vi "From String Array.vi"(8 "error in (no error)":errorcluster, 9 "String Array":string[](array[string]), 11 "Wait On Integer Step Config in":refnum<class "Wait On Integer Config.lvclass">) -> (0 "error out":errorcluster, 1 "Elements Left":string[](array[string]), 2 "Version":string, 3 "Wait On Integer Step Config out":refnum<class "Wait On Integer Config.lvclass">)   [LabVIEW 2018, in "Wait On Integer Config.lvclass"]
uses:
  Wait On Integer Config.lvclass
  <vilib>/NI/Tag Bus/tag/Data Type.ctl
  <vilib>/NI/Tag Bus Module Framework/channel/channel classification.ctl
  Wait On Integer Config.lvclass/Wait On Integer Config.ctl
  classes/Step/Config/Step Config.lvclass
  <vilib>/NI/Tag Bus Module Framework/channel/TBM channel.lvclass
  <vilib>/NI/Tag Bus/tag/tag descriptor.lvclass
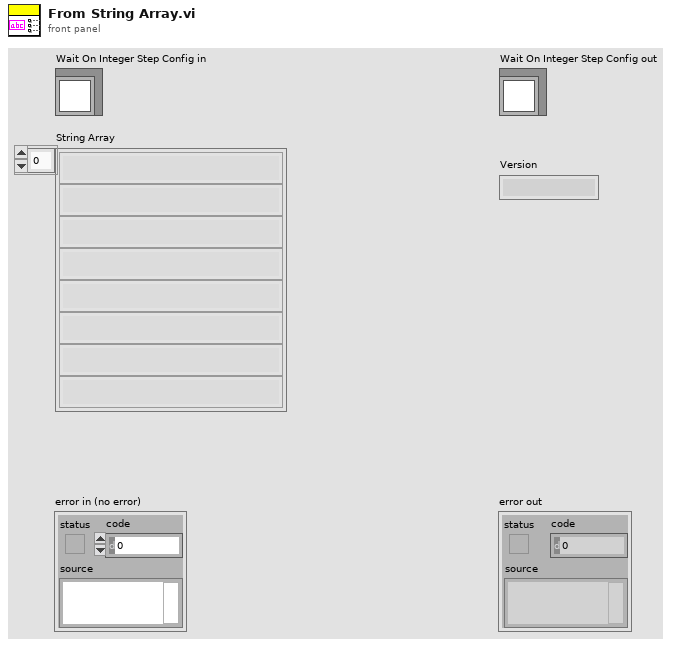
[diagram p1: front panel]
types:
  T1 = typedef "TBM channel.lvclass/channel classification.ctl" = enum16{"input data", "output data", "processing parameter", "processing result"}
  T2 = typedef "tag bus.lvlib/tag descriptor.lvclass/Data Type.ctl" = enum16{"Double", "Single", "I64", "I32", "I16", "I8", "U64", "U32", "U16", "U8", "Boolean", "String", "Array of Double", "Array of Single", "Array of I64", "Array of I32", "Array of I16", "Array of I8", "Array of U64", "Array of U32", "Array of U16", "Array of U8", "Array of Boolean", "Array of String"}
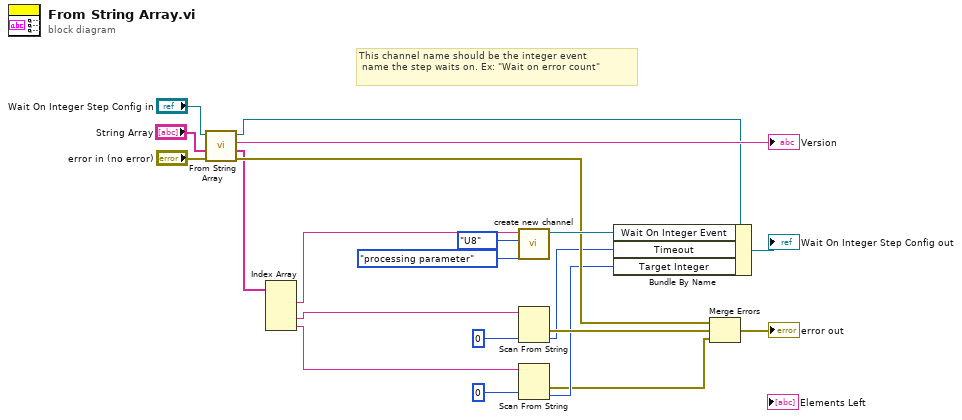
[diagram p0: block diagram]
diagram:
  # "This channel name should be the integer event\n name the step waits on. Ex: \"Wait on error count\""
  n1 = call-parent "From String Array.vi"("error in (no error)"="error in (no error)", "String Array"="String Array", "Step Config in"="Wait On Integer Step Config in") -> ("error out"=w11:errorcluster, "Elements Left"=w4:string[], "Version"=→"Version":string, "Step Config out"=w14:refnum<class "Wait On Integer Config.lvclass">)  [unwired: 5 in]
  n2 = Index Array(array=w4) -> (element #1=w3:string, element #3=w2:string, element #4=w1:string)  [unwired: 4 in, 1 out]
  n3 = call <vilib>:"create new channel.vi"("channel classification"=channel_classification."processing parameter", "data type"=Data_Type."U8", "channel name"=w3) -> ("channel"=w13:refnum<class "TBM channel.lvclass">)  [unwired: 8 in]
  n4 = Scan From String(input string=w2, default 1=0) -> (error out=w12:errorcluster, output 1=w8:i32)  [unwired: 3 in, 2 out]
  n5 = Scan From String(input string=w1, default 1=u32 0 ("Target Integer")) -> (error out=w5:errorcluster, output 1=w6:u32)  [unwired: 3 in, 2 out]
  n6 = Bundle By Name(cluster=w14, "Wait On Integer Event"=w13, "Timeout"=w8, "Target Integer"=w6) -> (→"Wait On Integer Step Config out":refnum<class "Wait On Integer Config.lvclass">)
  n7 = Merge Errors(w11, w12, w5) -> (→"error out":errorcluster)
